vi "OICB-get switches.vi"() -> (3 "Switch Inputs":T1)   [LabVIEW 2015]
uses:
  Projects/FRC Operator Interface Control Board/controlBoard_LabVIEW/Switch_Input_TypeDef.ctl
  <vilib>/Rock Robotics/Network Tables/NT Read Raw.vi
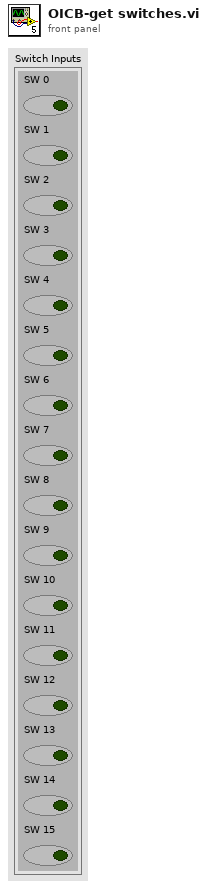
[diagram p1: front panel]
types:
  T1 = typedef "Switch_Input_TypeDef.ctl" = cluster{"SW 0":bool, "SW 1":bool, "SW 2":bool, "SW 3":bool, "SW 4":bool, "SW 5":bool, "SW 6":bool, "SW 7":bool, "SW 8":bool, "SW 9":bool, "SW 10":bool, "SW 11":bool, "SW 12":bool, "SW 13":bool, "SW 14":bool, "SW 15":bool}
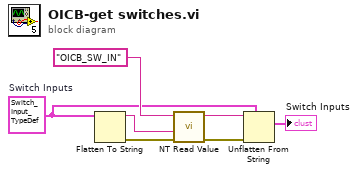
[diagram p0: block diagram]
diagram:
  w5 = T1 {"SW 0"=FALSE, "SW 1"=FALSE, "SW 2"=FALSE, "SW 3"=FALSE, "SW 4"=FALSE, "SW 5"=FALSE, "SW 6"=FALSE, "SW 7"=FALSE, "SW 8"=FALSE, "SW 9"=FALSE, "SW 10"=FALSE, "SW 11"=FALSE, "SW 12"=FALSE, "SW 13"=FALSE, "SW 14"=FALSE, "SW 15"=FALSE}  # Switch Inputs
  n1 = Flatten To String(anything=w5) -> (data string=w3:string, error out=w4:errorcluster)  [unwired: 3 in, 1 out]
  n2 = call-poly <vilib>:"NT Read Value.vi"("error in"=w4, "Default Value"=w3, "Name"="OICB_SW_IN") -> ("error out"=w2:errorcluster, "Raw"=w1:string)  [unwired: 7 in]
  n3 = Unflatten From String(type=w5, binary string=w1, error in (no error)=w2) -> (value=→"Switch Inputs":T1)  [unwired: 2 in, 2 out]
